vi "ConveyorBeltByValue_Init.vi"(0 "object in":refnum<class "ConveyorBeltByValue.lvclass">, 2 "ConveyorBeltRef":refnum<vi>, 5 "error in (no error)":errorcluster) -> (14 "object out":refnum<class "ConveyorBeltByValue.lvclass">, 19 "error out":errorcluster)   [LabVIEW 2014, in "ConveyorBeltByValue.lvclass"]
uses:
  ConveyorBeltByValue.lvclass
  ConveyorBeltByValue.lvclass/ConveyorBeltByValue.ctl
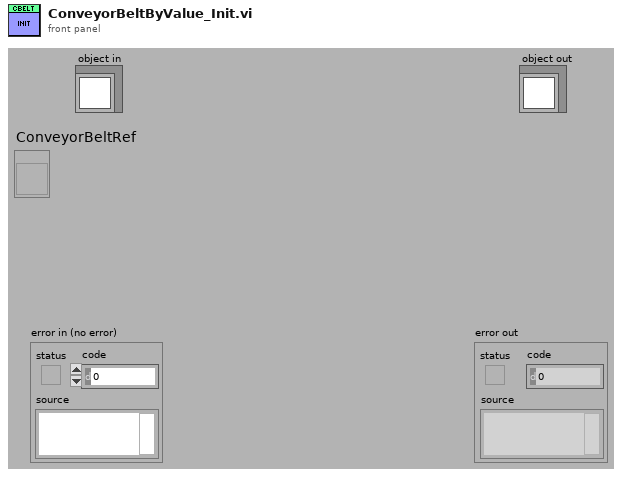
[diagram p1: front panel]
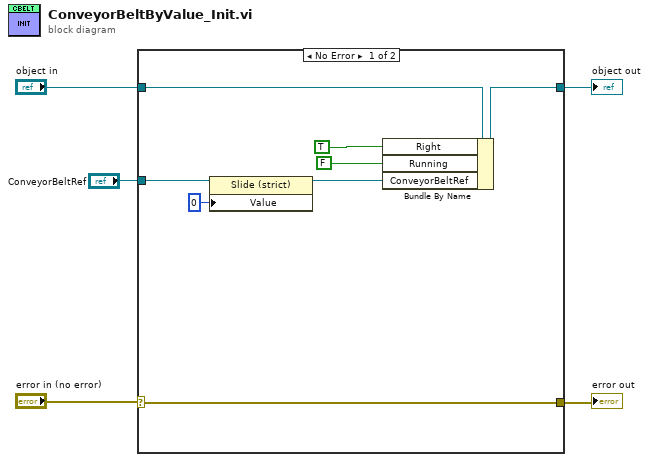
[diagram p0: block diagram]
diagram:
  n1 = case shown="No Error" "error in (no error)" {
    selector: "error in (no error)" -> [w10 w14]
    tunnel: "object in" -> [w13 w15]
    tunnel: [w12 w15] -> w4
    tunnel: [w10 w14] -> w2
    tunnel: "ConveyorBeltRef" -> [w8 _]
    frame No Error {
      n2 = property class="Slide (strict)"(reference=w8, "Value"=u8 0) -> (reference out=w7:refnum<vi>)  [unwired: 1 in, 1 out]
      n3 = Bundle By Name(cluster=w13, "Right"=TRUE ("None"), "Running"=FALSE, "ConveyorBeltRef"=w7) -> (w12:refnum<class "ConveyorBeltByValue.lvclass">)
    }
    frame Error {
    }
  }
  "object out" <- w4
  "error out" <- w2
